vi "Moving Average (single).vi"(6 "Window Unit (points)":enum16{"Points", "Data"}(ring), 8 "error in (no error)":errorcluster, 10 "Window":dbl, 11 "XY-data":cluster{"X-array":dbl[], "Y-array":dbl[]}) -> (0 "error out":errorcluster, 3 "XY-data out":cluster{"X-array":dbl[], "Y-array":dbl[]} {"Y-array" format="%.2p"; "X-array" format="%.2p"})   [LabVIEW 2019, in "xy_utilities.lvlib"]
doc: "Apply a moving average <b>XY-data</b>'s Y-Array according to <b>window</b>\n\nWire data to the data input to determine the polymorphic instance to use or manually select the instance."
uses:
  xy_utilities.lvlib
  Private/X Array Range to Index.vi
  Get X and Y.vi
  Get X and Y (single).vi
  Get Size (single).vi
  <vilib>/ptbypt/NI_PtbyPt.lvlib
  Circular Buffer (single).vi
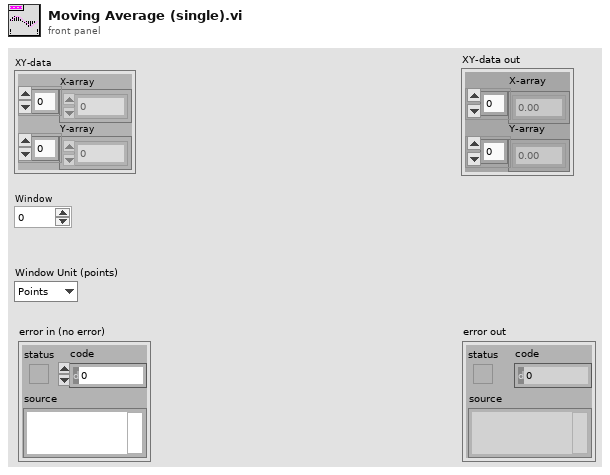
[diagram p1: front panel]
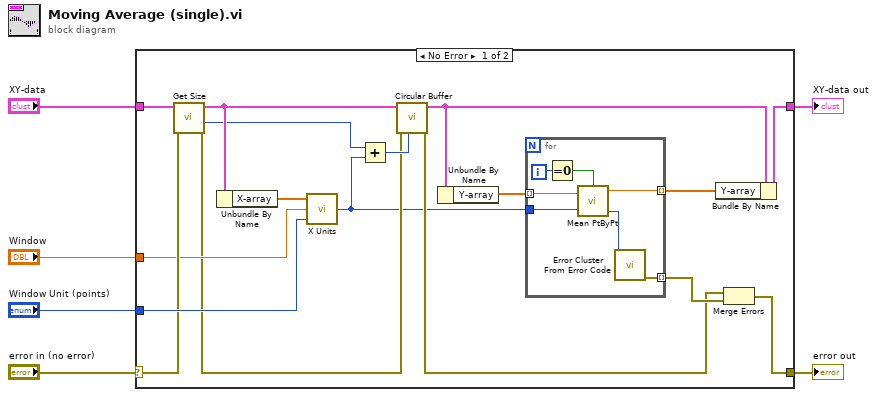
[diagram p0: block diagram]
diagram:
  n1 = case shown="No Error" "error in (no error)" {
    selector: "error in (no error)" -> [w16 w32]
    tunnel: [w21 w32] -> w5
    tunnel: "XY-data" -> [w15 w31]
    tunnel: [w23 w31] -> w3
    tunnel: "Window" -> [w14 _]
    tunnel: "Window Unit (points)" -> [w18 _]
    frame No Error {
      n2 = call-poly "Get Size.vi"("error in (no error)"=w16, "XY-data"=w15) -> ("error out"=w12:errorcluster, "X size"=w7:i32, "XY-data out"=w13:cluster{"X-array":dbl[], "Y-array":dbl[]})  [unwired: 6 in, 1 out]
      n3 = Unbundle By Name(w13) -> ("X-array"=w20:dbl[])
      n4 = call "X Units.vi"("Interval Units (points)"=w18, "Interval (h)"=w14, "X-array"=w20) -> ("h (points)"=w8:i32)
      n5 = Add(x=w7, y=w8) -> (x+y=w17:i32)
      n6 = call-poly "Circular Buffer.vi"("History Length [1024]"=w17, "error in"=w12, "XY-data"=w13) -> ("error out"=w11:errorcluster, "XY-data out"=w9:cluster{"X-array":dbl[], "Y-array":dbl[]})  [unwired: 7 in]
      n7 = Unbundle By Name(w9) -> ("Y-array"=w10:dbl[])
      n8 = for {
        tunnel: w10 -> [w30] mode=indexing
        tunnel: [w29] -> w22 mode=indexing
        tunnel: w8 -> [w28]
        tunnel: [w24] -> w19 mode=indexing
        i -> [w26]
        n9 = Equal To 0?(x=w26) -> (x = 0?=w27:bool)
        n10 = call <vilib>:"Mean PtByPt.vi"("x"=w30, "sample length"=w28, "initialize"=w27) -> ("mean"=w29:dbl, "error"=w25:i32)  [unwired: 1 in]
        n11 = call <vilib>:"Error Cluster From Error Code.vi"("error code (0)"=w25) -> ("error out"=w24:errorcluster)  [unwired: 8 in]
      }
      n12 = Bundle By Name(cluster=w9, "Y-array"=w22) -> (w23:cluster{"X-array":dbl[], "Y-array":dbl[]})
      n13 = Merge Errors(w11, w19) -> (w21:errorcluster)
    }
    frame Error {
    }
  }
  "error out" <- w5
  "XY-data out" <- w3
